vi "VdP4t.vi"() -> ()   [LabVIEW 2013]
panel:
  in  "VdP 4t Resistance":dbl
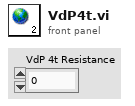
[diagram p1: front panel]
diagram:
